vi "Read DVR.vi"(8 "error in (no error)":errorcluster, 11 "Base Hardware in":refnum<class "Base Hardware.lvclass">) -> (0 "error out":errorcluster, 2 "DVR":refnum<data-value>, 3 "Base Hardware out":refnum<class "Base Hardware.lvclass">)   [LabVIEW 2023]
uses:
  Base Hardware.lvclass
  Base Hardware.lvclass/Base Hardware.ctl
  C:/Program Files/National Instruments/LabVIEW 2023/vi.lib/addons/_Workers/Library/Classes/Worker/Worker.lvclass
  C:/Program Files/National Instruments/LabVIEW 2023/vi.lib/addons/_Workers/Library/Classes/Workers Object/Workers Object.lvclass
  J:/Work/Cortech/KTM 1001/Workers Hardware/Workers/Base Classes/Base Hardware/Base Hardware.lvclass
  J:/Work/Cortech/KTM 1001/Workers Hardware/Hardware Interface/Hardware Interface.lvclass
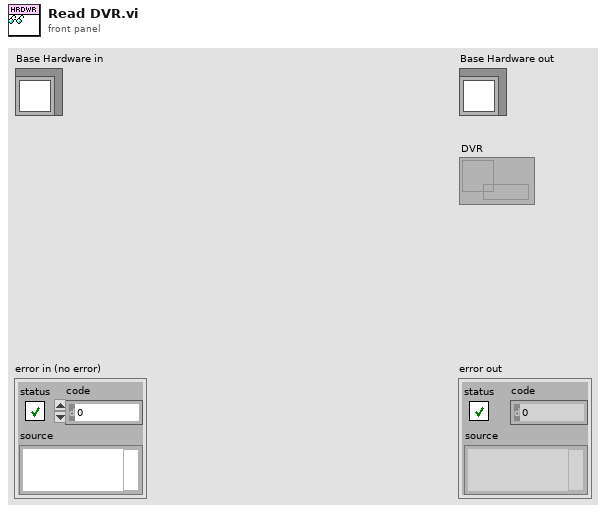
[diagram p1: front panel]
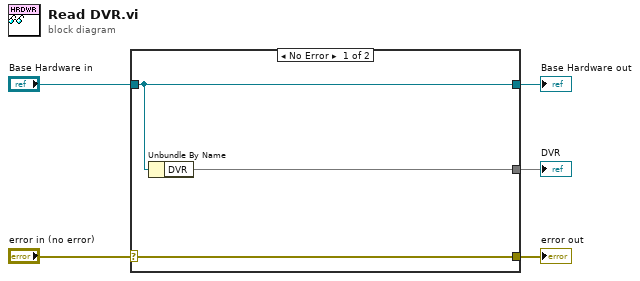
[diagram p0: block diagram]
diagram:
  n1 = case shown="No Error" "error in (no error)" {
    selector: "error in (no error)" -> [w8 w9]
    tunnel: [w8 w9] -> w4
    tunnel: [w7 w10] -> w2
    tunnel: "Base Hardware in" -> [w7 w10]
    tunnel: [w6 _] -> w1
    frame No Error {
      n2 = Unbundle By Name(w7) -> ("DVR"=w6)
    }
    frame Error {
    }
  }
  "error out" <- w4
  "Base Hardware out" <- w2
  "DVR" <- w1
